vi "Event Reg.vi"(11 "Builder in":refnum<class "Builder.lvclass">) -> (2 "Event Reg":refnum<event-registration>, 3 "Builder out":refnum<class "Builder.lvclass">)   [LabVIEW 2020, in "Builder Tools.lvlib" / "Builder.lvclass"]
uses:
  Builder.lvclass
  Builder.lvclass/Builder.ctl
  Enable Cancel Data.ctl
  Builder Tools.lvlib
  New Job Data.ctl
  New Item Data.ctl
  Complete Data.ctl
  Error Data.ctl
  Build Events.ctl
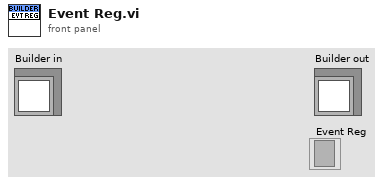
[diagram p1: front panel]
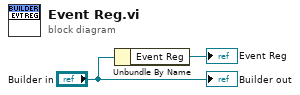
[diagram p0: block diagram]
diagram:
  n1 = Unbundle By Name("Builder in") -> ("Event Reg"=→"Event Reg":refnum<event-registration>)
  "Builder out" <- "Builder in"
